vi "From Pythonic - Boolean.vi"(4 "Pythonic Value":string) -> (1 "Boolean":bool)   [LabVIEW 2012, in "OPI.lvclass"]
doc: "Convert pythonic values into LabVIEW data. This method can be helpfull to convert elements of tuples or dictionaries.\n\nReturn a boolean."
uses:
  OPI.lvclass
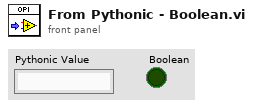
[diagram p1: front panel]
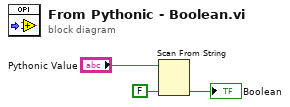
[diagram p0: block diagram]
diagram:
  n1 = Scan From String(input string="Pythonic Value", default 1=FALSE) -> (output 1=→"Boolean":bool)  [unwired: 3 in, 3 out]
